vi "PicoScope6000aaGetValuesBulk.vi"(5 "Segment Range":T1 {"toSegmentIndex" format="%.4p"; "fromSegmentIndex" format="%.4p"}, 7 "Buffer and Transfer Settings":T2 {"Down-Sample Mode" items=["None", "Aggregate", "Decimate", "Average"]; "Down Sample Ratio" step=1; "Samples" format="%_6p"}, 8 "error in (no error)":errorcluster, 11 "handle in":i16) -> (0 "error out":errorcluster, 3 "handle out":i16, 4 "overflow":i16[](array[numeric]) format="%010b", 6 "noOfSamples":u64)   [LabVIEW 2009]
doc: "Calls ps6000aGetValues"
uses:
  ps6000a.dll
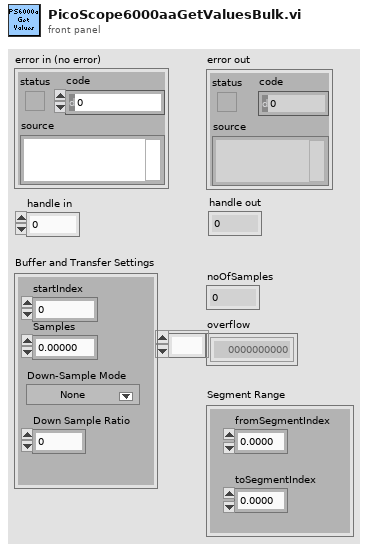
[diagram p1: front panel]
types:
  T1 = cluster{"fromSegmentIndex":u64, "toSegmentIndex":u64}
  T2 = cluster{"startIndex":u64, "Samples":u64, "Down Sample Ratio":u64, "Down-Sample Mode":u32}
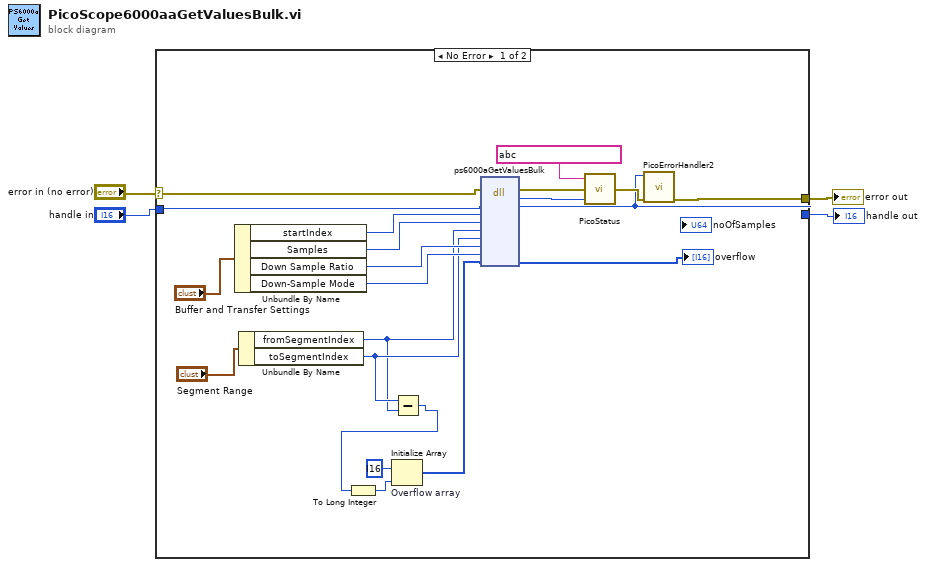
[diagram p0: block diagram]
diagram:
  n1 = case shown="No Error" "error in (no error)" {
    selector: "error in (no error)" -> [w8 w26]
    tunnel: "handle in" -> [w13 w27]
    tunnel: [w19 w27] -> w4
    tunnel: [w22 w26] -> w3
    frame #0 {
      n2 = Unbundle By Name("Buffer and Transfer Settings") -> ("startIndex"=w12:u64, "Samples"=w11:u64, "Down Sample Ratio"=w10:u64, "Down-Sample Mode"=w9:u32)
      n3 = Unbundle By Name("Segment Range") -> ("fromSegmentIndex"=w6:u64, "toSegmentIndex"=w7:u64)
      n4 = Subtract(x=w7, y=w6) -> (x-y=w14:u64)
      n5 = To Long Integer(number=w14) -> (32bit integer=w16:i32)
      n6 = Initialize Array "Overflow array"(i16 ? ("element"), w16) -> (w15:i16[])
      n7 = dll-call lib="ps6000a.dll" fn="ps6000aGetValuesBulk" ("ps3000.dll:_ps3000_open_unit@0")(error in=w8, "handle"=w13, "startIndex"=w12, "noOfSamples"=w11, "fromSegmentIndex"=w6, "toSegmentIndex"=w7, "downSampleRatio"=w10, "downSampleRatioMode"=w9, "overflow"=w15) -> (error out=w20:errorcluster, "PICO_STATUS"=w18:u32, "handle"=w19:i16, "overflow"=→"overflow":i16[])  [unwired: 8 in, 1 out]
      n8 = call "PicoStatus.vi"("PICO STATUS"=w18, "error in"=w20, "source"=string ?) -> ("error out"=w25:errorcluster)
      n9 = call "PicoErrorHandler2.vi"("error in (no error)"=w25, "handle In"=w19) -> ("error out"=w22:errorcluster)  [unwired: 9 in]
    }
    frame #1 {
    }
  }
  "error out" <- w3
  "handle out" <- w4
